vi "Release Blob Lease.vi"(6 "Lease ID":string, 8 "error in (no error)":errorcluster, 9 "Blob":string, 10 "Container":string, 11 "Azure Session in":refnum<class "Session.lvclass">) -> (0 "error out":errorcluster, 3 "Azure Session out":refnum<class "Session.lvclass">)   [LabVIEW 2015, in "NI_Azure_Blob.lvlib"]
doc: "Free the blob lease if it is no longer needed so that another client may immediately acquire a lease against the blob."
uses:
  NI_Azure_Blob.lvlib
  Core/Session/Session.lvclass
  Core/Name Value Pair.ctl
  Lease Action.ctl
  Core/Session/Session.lvclass/Session.ctl
  Core/Session/Write Request Headers.vi
  Core/Session/Write Request Parameters.vi
  Core/Session/Write HTTP Verb.vi
  Core/Session/Write URL Suffix.vi
  Core/NI_Azure_Core.lvlib
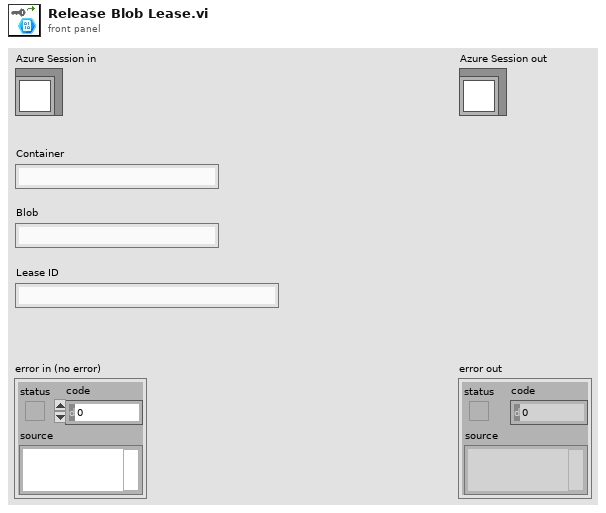
[diagram p1: front panel]
types:
  T1 = typedef "NI_Azure_Blob.lvlib/Lease Action.ctl" = enum16{"acquire", "renew", "change", "release", "break"}
  T2 = typedef "NI_Azure_Core.lvlib/Name Value Pair.ctl" = cluster{"name":string, "value":string}
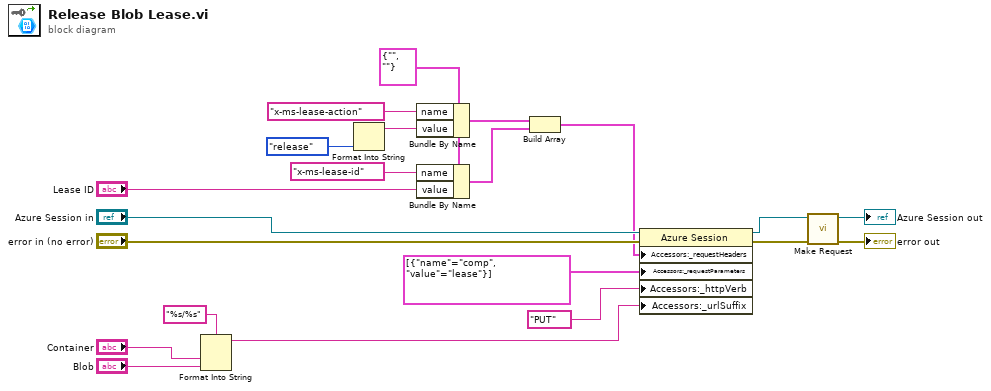
[diagram p0: block diagram]
diagram:
  w9 = T2 {"name"="", "value"=""} ("Cluster")
  n1 = Format Into String(format string="%s/%s", "Container", "Blob") -> (resulting string=w1:string)  [unwired: 2 in, 1 out]
  n2 = Format Into String(Lease_Action."release" ("Lease action")) -> (resulting string=w13:string)  [unwired: 3 in, 1 out]
  n3 = Bundle By Name(cluster=w9, "name"="x-ms-lease-action" ("header"), "value"=w13) -> (w15:T2)
  n4 = Bundle By Name(cluster=w9, "name"="x-ms-lease-id" ("header"), "value"="Lease ID") -> (w10:T2)
  n5 = Build Array(w15, w10) -> (w3:T2[])
  n6 = property class="Azure Session"(reference="Azure Session in", error in="error in (no error)", "Accessors:_requestHeaders"=w3, "Accessors:_requestParameters"=T2[] [{"name"="comp", "value"="lease"}] ("request parameters"), "Accessors:_httpVerb"="PUT" ("HTTP-Verb"), "Accessors:_urlSuffix"=w1) -> (reference out=w5:refnum<class "Session.lvclass">, error out=w7:errorcluster)
  n7 = call "Make Request.vi"("error in (no error)"=w7, "Session in"=w5) -> ("error out"=→"error out":errorcluster, "Session out"=→"Azure Session out":refnum<class "Session.lvclass">)  [unwired: 7 in, 1 out]
